vi "waitSweepStop.vi"(8 "error in (no error)":errorcluster, 11 "Instrument.Lockin in":refnum<class "Instrument.Lockin.lvclass">) -> (0 "error out":errorcluster, 3 "Instrument.Lockin out":refnum<class "Instrument.Lockin.lvclass">)   [LabVIEW 2016, in "Instrument.Lockin.lvclass"]
uses:
  Instrument.Lockin.lvclass
  Lockin.DAQ/Typedefs/State-enum.ctl
  Lockin.DAQ/Lockin.DAQ.lvclass
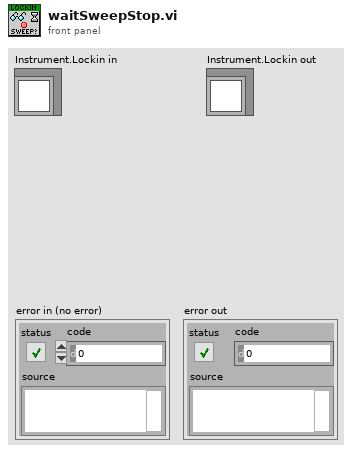
[diagram p1: front panel]
types:
  T1 = typedef "Lockin.DAQ.lvclass/State-enum.ctl" = enum16{"idle", "created", "started", "stopped", "sweeping"}
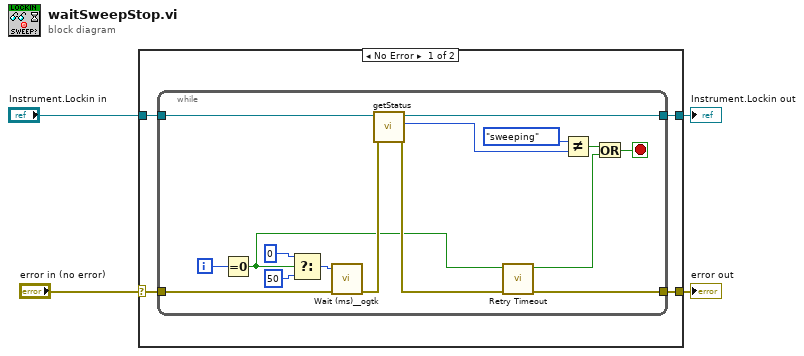
[diagram p0: block diagram]
diagram:
  n1 = case shown="No Error" "error in (no error)" {
    selector: "error in (no error)" -> [w5 w25]
    tunnel: [w8 w25] -> w4
    tunnel: [w7 w26] -> w3
    tunnel: "Instrument.Lockin in" -> [w6 w26]
    frame No Error {
      n2 = while {
        tunnel: w5 -> [w24]
        tunnel: [w13] -> w8
        tunnel: w6 -> [w19]
        tunnel: [w18] -> w7
        i -> [w11]
        stop <- w23 stop-if-true
        n3 = Equal To 0?(x=w11) -> (x = 0?=w10:bool)
        n4 = Select(t=u32 0, s=w10, f=u32 50 ("milliseconds to wait")) -> (s? t:f=w20:u32)
        n5 = call <userlib>:"Wait (ms)__ogtk.vi"("error in (no error)"=w24, "milliseconds to wait"=w20) -> ("error out"=w14:errorcluster)  [unwired: 8 in, 1 out]
        n6 = call "getStatus.vi"("error in (no error)"=w14, "Instrument.Lockin"=w19) -> ("error out"=w12:errorcluster, "Status"=w16:T1, "Instrument.Lockin"=w18:refnum<class "Instrument.Lockin.lvclass">)  [unwired: 7 in]
        n7 = call "Retry Timeout.vi"("error in (no error)"=w12, "reset"=w10) -> ("error out"=w13:errorcluster, "Timeout?"=w9:bool)  [unwired: 8 in]
        n8 = Not Equal?(x=State-enum."sweeping" ("Status"), y=w16) -> (x != y?=w15:bool)
        n9 = Or(x=w15, y=w9) -> (x .or. y?=w23:bool)
      }
    }
    frame Error {
    }
  }
  "error out" <- w4
  "Instrument.Lockin out" <- w3
